vi "AOC1_Part1_Template.vi"() -> ()   [LabVIEW 2015]
panel:
  out "Floor Number":i32
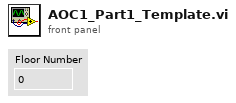
[diagram p1: front panel]
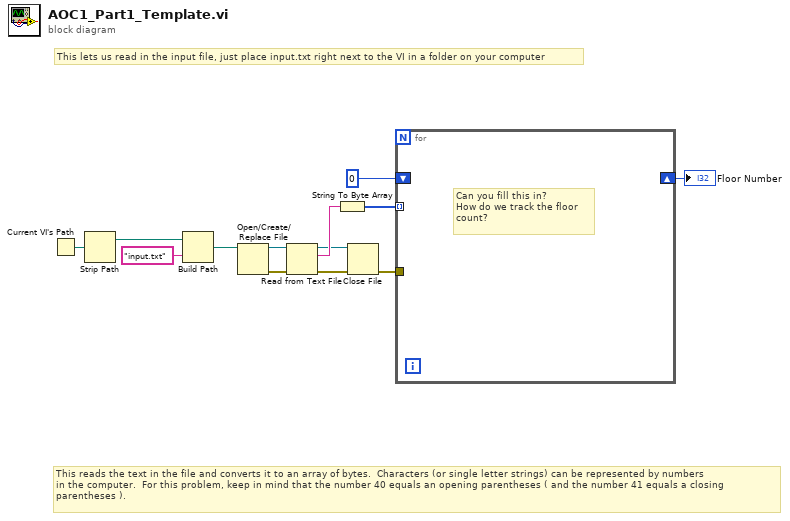
[diagram p0: block diagram]
diagram:
  # "This reads the text in the file and converts it to an array of bytes.  Characters (or single letter strings) can be represented by numbers\nin the computer.  For this problem, keep in mind that the number 40 equals an opening parentheses ( and the number 41 equals a closing\nparentheses )."
  # "This lets us read in the input file, just place input.txt right next to the VI in a folder on your computer"
  n1 = Current VI's Path() -> (path=w11:path)
  n2 = Strip Path(path=w11) -> (stripped path=w10:path)  [unwired: 1 out]
  n3 = Build Path(base path=w10, name or relative path="input.txt") -> (appended path=w8:path)
  n4 = Open/Create/Replace File(file path (use dialog)=w8) -> (refnum out=w12:refnum<file>, error out=w13:errorcluster)  [unwired: 5 in, 1 out]
  n5 = Read from Text File(file (use dialog)=w12, error in=w13) -> (refnum out=w5:refnum<file>, text=w7:string, error out=w6:errorcluster)  [unwired: 2 in, 1 out]
  n6 = String To Byte Array(string=w7) -> (unsigned byte array=w4:u8[])
  n7 = Close File(refnum=w5, error in=w6) -> (error out=w3:errorcluster)  [unwired: 1 out]
  n8 = for {
    tunnel: w4 -> [_] mode=indexing
    tunnel: w3 -> [_]
    shift-right: [_] -> w1
    shift-left: 0 -> [_]
    # "Can you fill this in?\nHow do we track the floor\ncount?"
  }
  "Floor Number" <- w1
